vi "test_Equal_dbl.vi"(8 "error in (no error)":errorcluster, 11 "TestCase in":refnum<class "Equals Test.lvclass">) -> (0 "error out":errorcluster, 3 "TestCase out":refnum<class "Equals Test.lvclass">)   [LabVIEW 2018, in "Equals Test.lvclass"]
uses:
  Equals Test.lvclass
  4713f549-16d3-4bca-b5d1-e772303f63ef.vi
  48e687d7-bb32-45f7-8012-851ac34d1ce8.vi
  f1ce6a55-5bee-417f-b038-942a6de9ea27.vi
  2a0265de-d45e-4775-a441-dab26ac7cf19.vi
  4713f549-16d3-4bca-b5d1-e772303f63ef.vi/c42fa6df-0fa9-4903-a255-79594b42ba5a.vi
  48e687d7-bb32-45f7-8012-851ac34d1ce8.vi/fe9b554d-a228-4b24-b6f1-8ce6c9e59a8e.vi
  f1ce6a55-5bee-417f-b038-942a6de9ea27.vi/11c88adb-2574-4210-9fbf-a4828fd58ec4.vi
  2a0265de-d45e-4775-a441-dab26ac7cf19.vi/ca83ea39-fae0-45fe-9423-4ea14323f7c0.vi
  <vilib>/addons/_JKI Toolkits/VI Tester/TestCase.llb/TestCase.lvclass
  C:/Program Files (x86)/National Instruments/LabVIEW 2018/vi.lib/addons/_JKI Toolkits/VI Tester/TestCase.llb/TestCase.lvclass
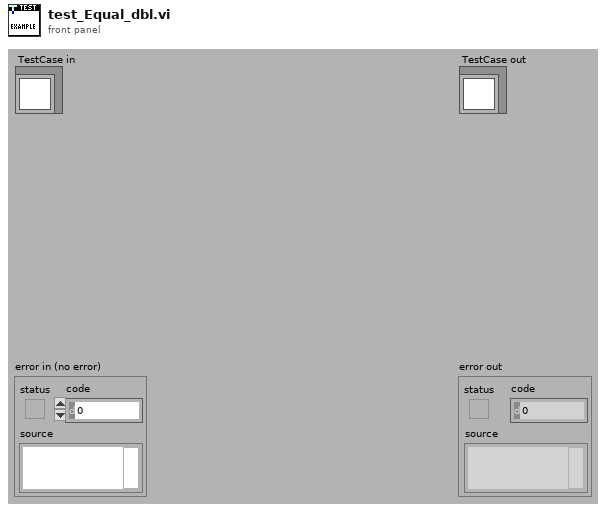
[diagram p1: front panel]
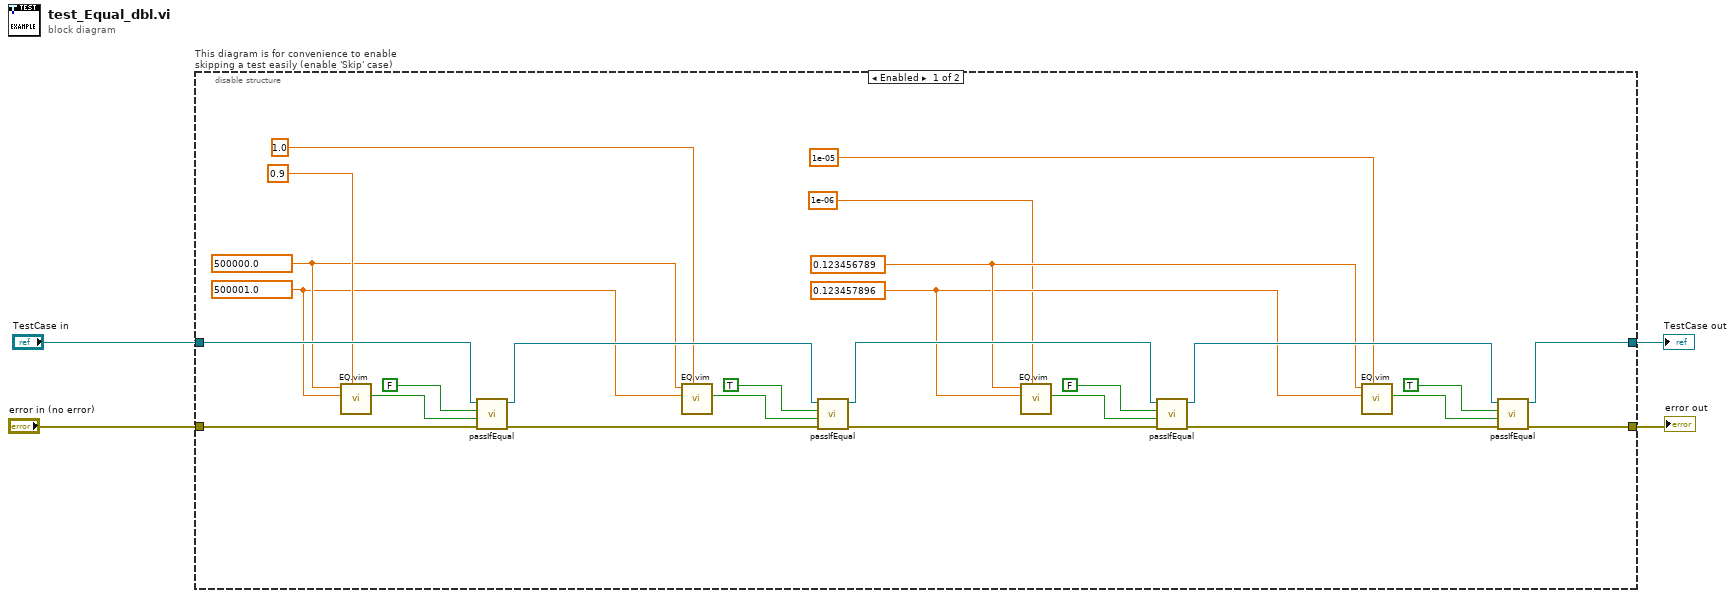
[diagram p0: block diagram]
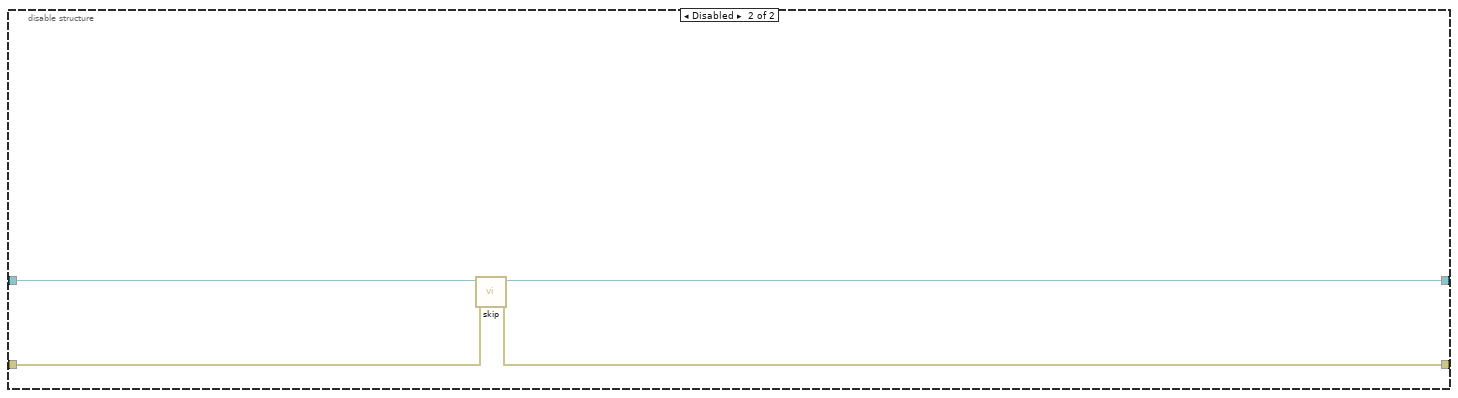
[diagram p2: hidden frame]
diagram:
  n1 = disable-structure "This diagram is for convenience to enable skipping a test easily (enable 'Skip' case)" shown="Enabled" {
    disable-tunnel: "TestCase in" -> [w30 w34]
    disable-tunnel: [w13 w32] -> w1
    disable-tunnel: [w15 w33] -> w3
    disable-tunnel: "error in (no error)" -> [w29 w31]
    frame Enabled {
      w10 = 0.123457896 ("x")
      w11 = 0.123456789 ("x")
      w7 = 500001.0 ("x")
      w8 = 500000.0 ("x")
      n2 = call "EQ.vim"("Relative Epsilon"=0.9 ("Required Digits of Precision"), "y"=w7, "x"=w8) -> ("Equal?"=w28:bool)  [unwired: 8 in]
      n3 = call-dynamic "passIfEqual.vi"("error in (no error)"=w29, "y"=w28, "x"=FALSE, "TestCase in"=w30) -> ("error out"=w24:errorcluster, "TestCase out"=w23:refnum<class "Equals Test.lvclass">)  [unwired: 6 in]
      n4 = call "EQ.vim"("Relative Epsilon"=1.0 ("Required Digits of Precision"), "y"=w7, "x"=w8) -> ("Equal?"=w25:bool)  [unwired: 8 in]
      n5 = call-dynamic "passIfEqual.vi"("error in (no error)"=w24, "y"=w25, "x"=TRUE, "TestCase in"=w23) -> ("error out"=w16:errorcluster, "TestCase out"=w14:refnum<class "Equals Test.lvclass">)  [unwired: 6 in]
      n6 = call "EQ.vim"("Relative Epsilon"=1e-06, "y"=w10, "x"=w11) -> ("Equal?"=w17:bool)  [unwired: 8 in]
      n7 = call-dynamic "passIfEqual.vi"("error in (no error)"=w16, "y"=w17, "x"=FALSE, "TestCase in"=w14) -> ("error out"=w21:errorcluster, "TestCase out"=w22:refnum<class "Equals Test.lvclass">)  [unwired: 6 in]
      n8 = call "EQ.vim"("Relative Epsilon"=1e-05, "y"=w10, "x"=w11) -> ("Equal?"=w20:bool)  [unwired: 8 in]
      n9 = call-dynamic "passIfEqual.vi"("error in (no error)"=w21, "y"=w20, "x"=TRUE, "TestCase in"=w22) -> ("error out"=w15:errorcluster, "TestCase out"=w13:refnum<class "Equals Test.lvclass">)  [unwired: 6 in]
    }
    frame Disabled {
      # "skip test result while test is under development"
      n10 = call <vilib>:"skip.vi"("error in (no error)"=w31, "TestCase in"=w34) -> ("error out"=w33:errorcluster, "TestCase out"=w32:refnum<class "Equals Test.lvclass">)  [unwired: 8 in]
    }
  }
  "error out" <- w3
  "TestCase out" <- w1
